vi "iWorx - Event Marker.vi"() -> ()   [LabVIEW 2012]
uses:
  <vilib>/DAQmx/create/channels.llb/DAQmx Create Channel (AI-Voltage-Basic).vi
  <vilib>/DAQmx/configure/timing.llb/DAQmx Timing (Sample Clock).vi
  <vilib>/DAQmx/read.llb/DAQmx Read (Analog 1D Wfm NChan NSamp).vi
panel:
  in  "Stop":bool
  out "Button Press Durration":dbl format="%.3f"
  in  "Set Up":bool
  out "Waveform Chart":waveform(dbl)(graph)
  in  "Snapshot":bool
  in  "Pause Button":bool
  in  "Clear Chart":bool
  out "Button Press Delta t":dbl format="%.3f"
  out "Button Press Count":u32
  in  "Reset Counter":bool
  out "Button Pressed":bool
  in  "Channel":u16(ring) items=["Channel 1", "Channel 2"]
  # "iWorx - Event Marker - Data Logger"
  # "Sensor Input"
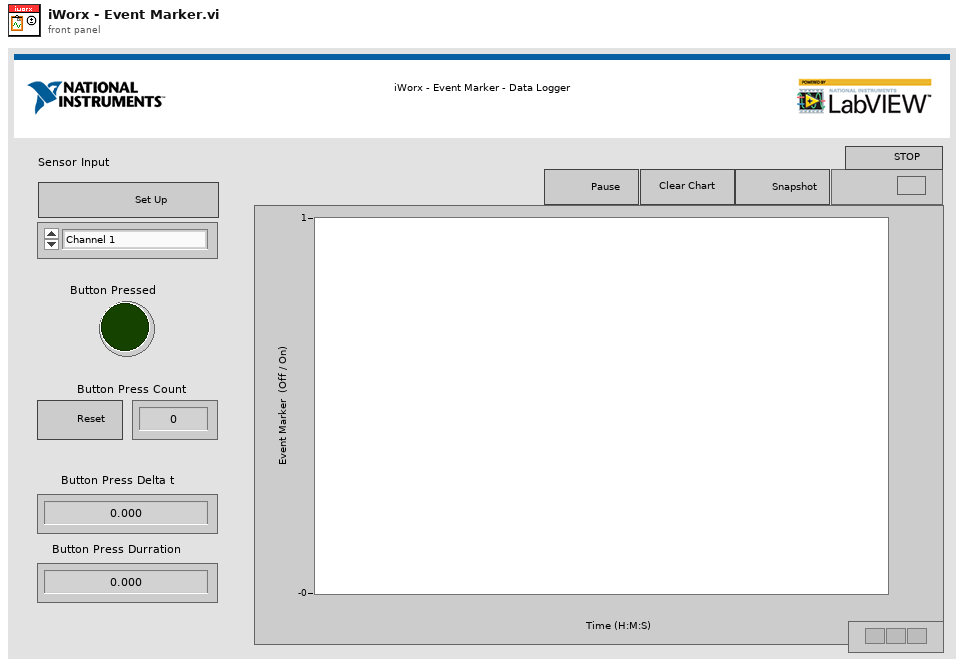
[diagram p1: front panel]
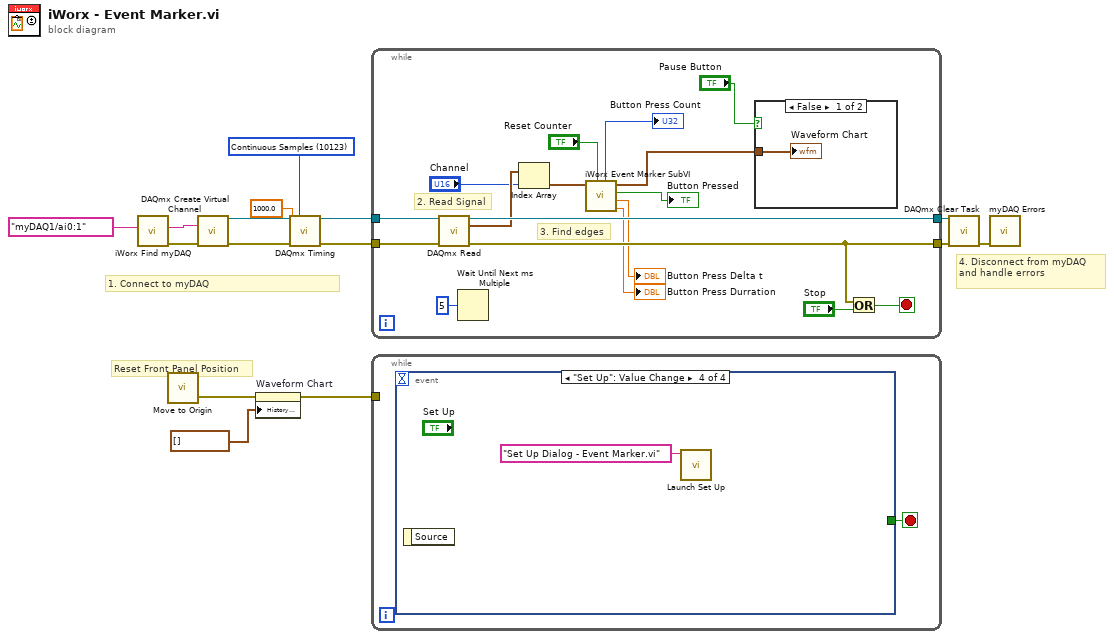
[diagram p0: block diagram]
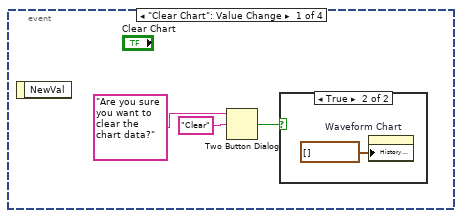
[diagram p2: hidden frame]
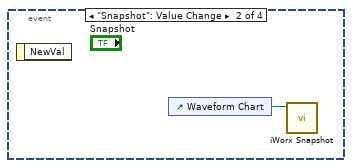
[diagram p4: hidden frame]
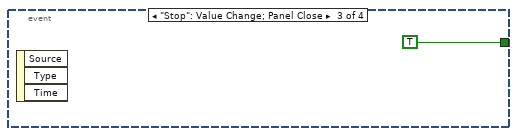
[diagram p5: hidden frame]
diagram:
  w9 = 10123 items=["Finite Samples"=10178, "Continuous Samples"=10123, "Hardware Timed Single Point"=12522] ("sample mode")
  # "Reset Front Panel Position"
  # "4. Disconnect from myDAQ and handle errors"
  # "1. Connect to myDAQ"
  n1 = call "iWorx Find myDAQ.vi"("Preferred myDAQ (myDAQ1)"=tag "myDAQ1/ai0:1" ("physical channels")) -> ("Error Out"=w2:errorcluster, "DAQmx Physical Channel"=w3:tag)  [unwired: 6 in, 3 out]
  n2 = call "Move to Origin.vi"() -> ("Error Out"=w1:errorcluster)  [unwired: 3 in]
  n3 = call-poly <vilib>:"DAQmx Create Virtual Channel.vi"("physical channels"=w3, "error in"=w2) -> ("task out"=w13:refnum<k21>, "error out"=w7:errorcluster)  [unwired: 12 in]
  n4 = property on="Waveform Chart" class="WFChart (strict)"(error in=w1, "History Data"=waveform(dbl)[] []) -> (error out=w12:errorcluster)  [unwired: 1 in, 1 out]
  n5 = call-poly <vilib>:"DAQmx Timing.vi"("task/channels in"=w13, "sample mode"=w9, "rate"=1000.0, "error in"=w7) -> ("task out"=w10:refnum<k21>, "error out"=w6:errorcluster)  [unwired: 10 in]
  n6 = while {
    tunnel: w10 -> [w32]
    tunnel: [w31] -> w15
    tunnel: w6 -> [w30]
    tunnel: [w28] -> w14
    stop <- w29 stop-if-true
    # "3. Find edges"
    # "2. Read Signal"
    n7 = call-poly <vilib>:"DAQmx Read.vi"("task/channels in"=w32, "error in"=w30) -> ("task out"=w31:refnum<k21>, "data"=w26:waveform(dbl)[], "error out"=w28:errorcluster)  [unwired: 11 in]
    n8 = Wait Until Next ms Multiple(millisecond multiple=u32 5) -> ()  [unwired: 1 out]
    n9 = Index Array(array=w26, index="Channel") -> (element=w16:waveform(dbl))
    n10 = call "iWorx Event Marker SubVI.vi"("Reset count (f)"="Reset Counter", "waveform in"=w16) -> ("Button Press Duration"=→"Button Press Durration":dbl, "Two Edge Separation (rising)"=→"Button Press Delta t":dbl, "Button State"=→"Button Pressed":bool, "0-1 Waveform out"=w23:waveform(dbl), "Button Count"=→"Button Press Count":u32)  [unwired: 3 in, 2 out]
    n11 = case shown="False" "Pause Button" {
      tunnel: w23 -> [w33 _]
      frame False {
        "Waveform Chart" <- w33
      }
      frame True {
      }
    }
    n12 = Or(x=w28, y="Stop") -> (x .or. y?=w29:bool)
  }
  n13 = while {
    tunnel: w12 -> [_]
    stop <- w34 stop-if-true
    n14 = event shown="[3] \"Set Up\": Value Change" {
      selector: _ -> [_ _ _ _]
      dyn-events: _ -> [_ _ _ _]
      timeout: _ -> [_ _ _ _]
      tunnel: [_ _ TRUE _] -> w34
      event "Clear Chart": Value Change {
        n15 = event-data() -> ()  [unwired: 1 in, 1 out]
        n16 = Two Button Dialog(message="Are you sure you want to clear the chart data?", 2:"Clear" ("T button name (\"OK\")")) -> (T button?=w36:bool)  [unwired: 1 in]
        n17 = case shown="True" w36 {
          frame False {
          }
          frame True {
            n18 = property on="Waveform Chart" class="WFChart (strict)"("History Data"=waveform(dbl)[] []) -> ()  [unwired: 2 in, 2 out]
          }
        }
      }
      event "Snapshot": Value Change {
        n19 = event-data() -> ()  [unwired: 1 in, 1 out]
        n20 = control-ref of="Waveform Chart"() -> (w39:refnum<vi>)
        n21 = call "iWorx Snapshot.vi"("WaveformChart in"=w39) -> ()  [unwired: 10 in, 1 out]
      }
      event "Stop": Value Change; Panel Close {
        n22 = event-data() -> ()  [unwired: 1 in, 3 out]
      }
      event "Set Up": Value Change {
        n23 = event-data() -> ()  [unwired: 1 in, 1 out]
        n24 = call "Launch Set Up.vi"("name or relative path"="Set Up Dialog - Event Marker.vi") -> ()  [unwired: 9 in, 2 out]
      }
    }
  }
  n25 = call <vilib>:"DAQmx Clear Task.vi"("task in"=w15, "error in"=w14) -> ("error out"=w5:errorcluster)  [unwired: 13 in]
  n26 = call "myDAQ Errors.vi"("error in (no error)"=w5) -> ()  [unwired: 10 in, 1 out]
